vi "Find VI with Focus.vi"(8 "error in":errorcluster caption="error in (no error)", 9 "Exclude Callers":bool=TRUE caption="Exclude All Callers (T)", 10 "Exclude Levels":i32=-1 caption="Exclude Levels (call chain=-1)", 11 "Exclude Names":string[](array[string]) caption="Exclude Names (none)") -> (0 "error out":errorcluster, 1 "Changed?":bool, 2 "VI with Focus":refnum<vi>, 3 "Valid?":bool, 5 "VI Name":string)   [LabVIEW 2020]
doc: "Returns a reference to the frontmost VI panel. \n\nThis VI is reentrant (as indicated by the crosshatched background) so that references in use by one caller aren't closed by another. This also allows different callers to exclude different panels from consideration and to get a proper indication of whether a changed has occurred since their own last last call.\n\nThis is an enhancement of Jim Kring's Find Frontmost VI that returns a reference as well as a name, signals if this has changed since the last call, allows exclusion of VIs in the calling sequence of this VI or other VIs of the user's choice (useful for editing utilities that stay on top of all other windows), cleans up unused references, and runs, on average, 50 or more times faster.\n\nGenerates no errors.\n\nCopyright © 2003 by Paul F. Sullivan. All rights reserved. You are only permitted the usage indicated in your license agreement."
uses:
  TypeDefs/Find Focus State.ctl
panel:
  out "State Data":T2={"State"=enum."Excluded?", "Recent VI"=refnum, "Recent Number"=0, "Recent VI Name"="", "VI with Focus"=refnum, "Focus Number"=0, "Focus VI Name"="", "Valid?"=FALSE, "Changed?"=FALSE} {"Focus Number" format="%.0x"; "Recent Number" format="%.0x"}
  in  "State Data":T2={"State"=enum."Recent?", "Recent VI"=refnum, "Recent Number"=0, "Recent VI Name"="", "VI with Focus"=refnum, "Focus Number"=0, "Focus VI Name"="", "Valid?"=FALSE, "Changed?"=FALSE} {"Focus Number" format="%.0x"; "Recent Number" format="%.0x"}
  # "Find VI with Focus.vi\n\nReturns a reference to the frontmost VI panel.\n\nPlease visit http://www.OpenG.org to learn about the\nOpen Source LabVIEW software movement.\n\nNOTICE -- YOU MUST LEAVE THIS NOTICE IN PLACE.  PER THE TERMS OF THE LICENSE BELOW, YOU MAY SUBLICENSE THIS SOFTWARE \nIN ANY WAY THAT DOES NOT CONFLICT WITH THIS LICENSE.\n\n### BSD License (http://www.opensource.org/licenses/bsd-license.php) Begin ###\n \nCopyright (c) 2003, Paul F. Sullivan <Paul@SULLutions.com>\n\nAll rights reserved.\n\nRedistribution and use in source and binary forms, with or without modification, are permitted provided that the following conditions are met:\n\n    * Redistributions of source code must retain the above copyright notice, this list of conditions and the following disclaimer.\n    * Redistributions in binary form must reproduce the above copyright notice, this list of conditions and the following disclaimer in the \n       documentation and/or other materials provided with the distribution.\n    * Neither the name of SciWare, James Kring, Inc., nor the names of its contributors may be used to endorse or promote products derived \n       from this software without specific prior written permission.\n\nTHIS SOFTWARE IS PROVIDED BY THE COPYRIGHT HOLDERS AND CONTRIBUTORS \"AS IS\" AND ANY EXPRESS OR IMPLIED WARRANTIES, \nINCLUDING, BUT NOT LIMITED TO, THE IMPLIED WARRANTIES OF MERCHANTABILITY AND FITNESS FOR A PARTICULAR PURPOSE ARE \nDISCLAIMED. IN NO EVENT SHALL THE COPYRIGHT OWNER OR CONTRIBUTORS BE LIABLE FOR ANY DIRECT, INDIRECT, INCIDENTAL,\n SPECIAL, EXEMPLARY, OR CONSEQUENTIAL DAMAGES (INCLUDING, BUT NOT LIMITED TO, PROCUREMENT OF SUBSTITUTE GOODS OR \nSERVICES; LOSS OF USE, DATA, OR PROFITS; OR BUSINESS INTERRUPTION) HOWEVER CAUSED AND ON ANY THEORY OF LIABILITY, \nWHETHER IN CONTRACT, STRICT LIABILITY, OR TORT (INCLUDING NEGLIGENCE OR OTHERWISE) ARISING IN ANY WAY OUT OF THE USE \nOF THIS SOFTWARE, EVEN IF ADVISED OF THE POSSIBILITY OF SUCH DAMAGE.\n\n### BSD License End ###"
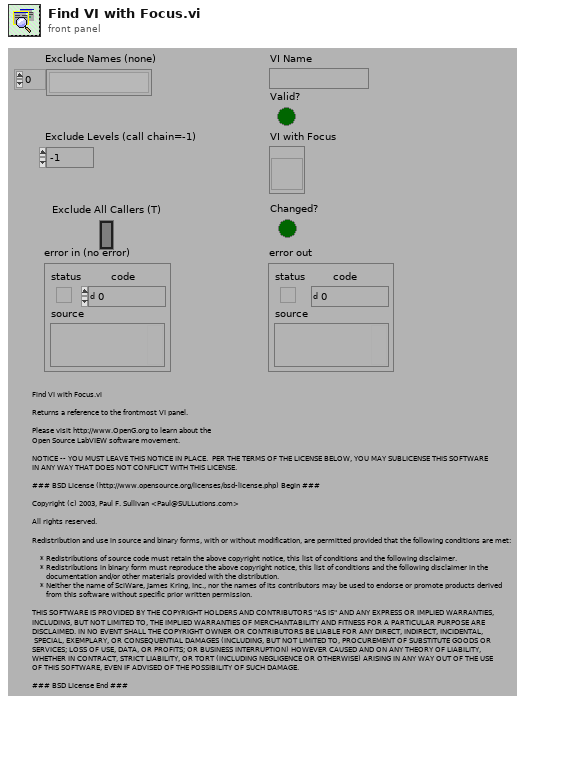
[diagram p1: front panel]
types:
  T1 = typedef "Find Focus State.ctl" = enum16{"Initialize", "Recent?", "Accepted?", "Excluded?", "VI Panel?", "Valid?", "Done"}
  T2 = cluster{"State":T1, "Recent VI":refnum<vi>, "Recent Number":u32, "Recent VI Name":string, "VI with Focus":refnum<vi>, "Focus Number":u32, "Focus VI Name":string, "Valid?":bool, "Changed?":bool}
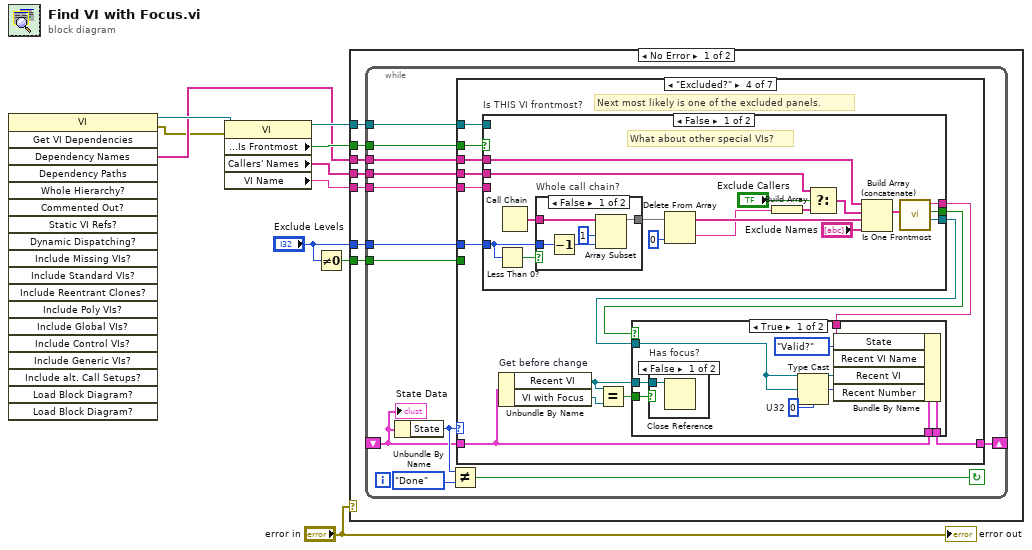
[diagram p0: block diagram]
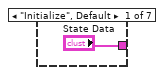
[diagram p2: hidden frame]
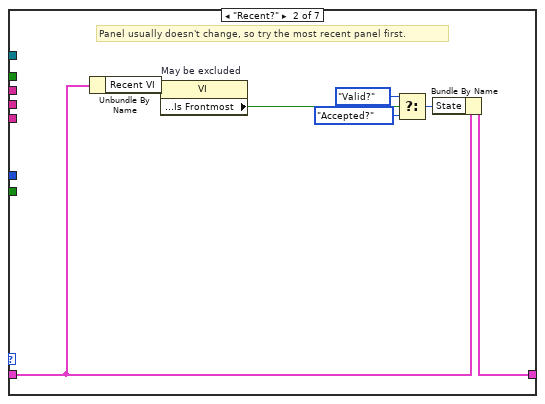
[diagram p3: hidden frame]
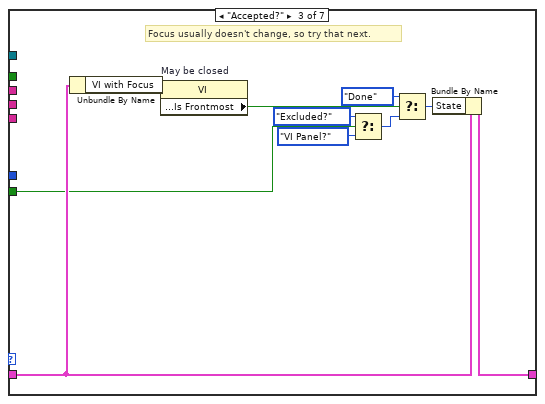
[diagram p4: hidden frame]
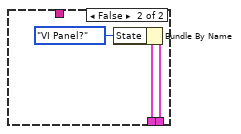
[diagram p6: hidden frame]
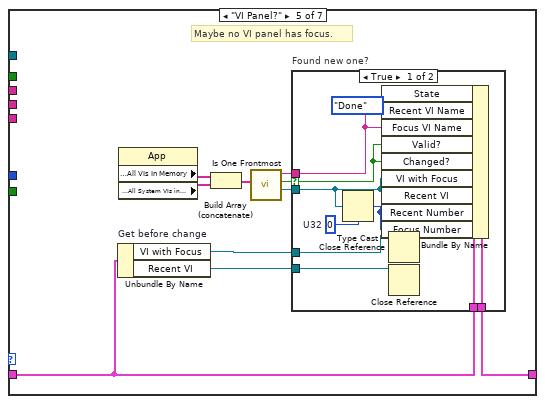
[diagram p9: hidden frame]
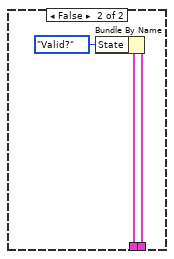
[diagram p10: hidden frame]
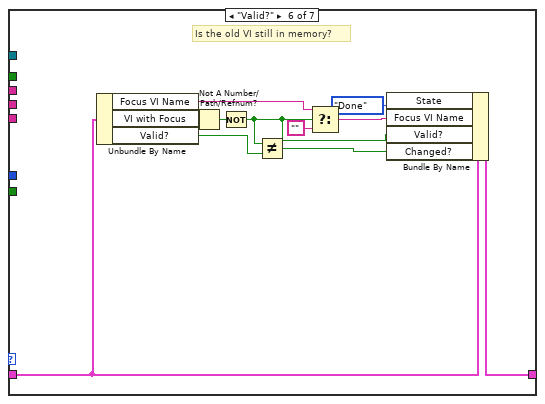
[diagram p11: hidden frame]
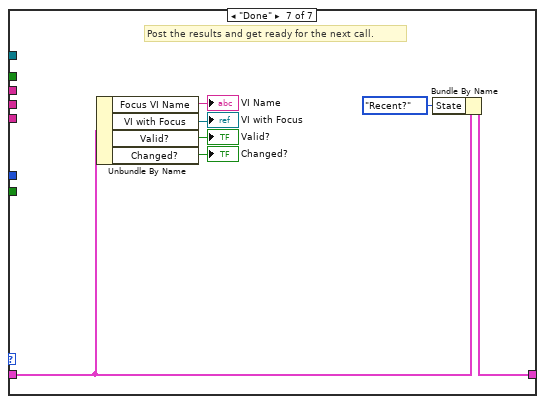
[diagram p12: hidden frame]
diagram:
  n1 = invoke class="VI" method="Get VI Dependencies"() -> (reference out=w3:refnum<vi>, error out=w1:errorcluster, "Dependency Names"=w2:string[])  [unwired: 19 in, 16 out]
  n2 = property class="VI"(reference=w3, error in=w1) -> (reference out=w7:refnum<vi>, "Front Panel Window:Is Frontmost"=w8:bool, "Callers' Names"=w9:string[], "VI Name"=w4:string)  [unwired: 1 out]
  n3 = Not Equal To 0?(x="Exclude Levels") -> (x != 0?=w5:bool)
  n4 = case shown="No Error" "error in" {
    tunnel: w9 -> [w17 _]
    tunnel: w2 -> [w16 _]
    tunnel: w8 -> [w15 _]
    tunnel: w7 -> [w14 _]
    tunnel: "Exclude Levels" -> [w13 _]
    tunnel: w5 -> [w12 _]
    tunnel: w4 -> [w11 _]
    frame No Error {
      n5 = while {
        tunnel: w11 -> [w19]
        tunnel: w12 -> [w21]
        tunnel: w13 -> [w22]
        tunnel: w14 -> [w20]
        tunnel: w15 -> [w23]
        tunnel: w16 -> [w24]
        tunnel: w17 -> [w25]
        shift-left: _ -> [w18]
        shift-right: [w27] -> _
        stop <- w26 continue-if-true
        n6 = Unbundle By Name(w18) -> ("State"=w28:T1)
        n7 = Not Equal?(x=w28, y=Find_Focus_State."Done" ("State")) -> (x != y?=w26:bool)
        n8 = case shown="\"Excluded?\"" w28 {
          tunnel: w23 -> [_ _ _ w61 _ _ _]
          tunnel: w25 -> [_ _ _ w60 _ _ _]
          tunnel: w24 -> [_ _ _ w59 _ _ _]
          tunnel: w22 -> [_ _ _ w58 _ _ _]
          tunnel: w21 -> [_ _ w39 _ _ _ _]
          tunnel: w18 -> [_ w36 w46 w51 w101 w131 w138]
          tunnel: ["State Data" w35 w45 w57 w106 w130 w137] -> w27
          tunnel: w20 -> [_ _ _ w54 _ _ _]
          tunnel: w19 -> [_ _ _ w52 _ _ _]
          frame "Initialize", Default {
          }
          frame "Recent?" {
            # "Panel usually doesn't change, so try the most recent panel first."
            n9 = Unbundle By Name(w36) -> ("Recent VI"=w37:refnum<vi>)
            n10 = property on="May be excluded" class="VI"(reference=w37) -> ("Front Panel Window:Is Frontmost"=w33:bool)  [unwired: 1 in, 2 out]
            n11 = Select(t=Find_Focus_State."Valid?" ("State"), s=w33, f=Find_Focus_State."Accepted?" ("State")) -> (s? t:f=w34:T1)
            n12 = Bundle By Name(cluster=w36, "State"=w34) -> (w35:T2)
          }
          frame "Accepted?" {
            # "Focus usually doesn't change, so try that next."
            n13 = Unbundle By Name(w46) -> ("VI with Focus"=w47:refnum<vi>)
            n14 = property on="May be closed" class="VI"(reference=w47) -> ("Front Panel Window:Is Frontmost"=w43:bool)  [unwired: 1 in, 2 out]
            n15 = Select(t=Find_Focus_State."Excluded?" ("State"), s=w39, f=Find_Focus_State."VI Panel?" ("State")) -> (s? t:f=w40:T1)
            n16 = Select(t=Find_Focus_State."Done" ("State"), s=w43, f=w40) -> (s? t:f=w44:T1)
            n17 = Bundle By Name(cluster=w46, "State"=w44) -> (w45:T2)
          }
          frame "Excluded?" {
            # "Next most likely is one of the excluded panels."
            n18 = case "Is THIS VI frontmost?" shown="False" w61 {
              selector: w61 -> [_ w100]
              tunnel: w58 -> [w78 _]
              tunnel: [w77 w100] -> w56
              tunnel: w60 -> [w87 _]
              tunnel: w59 -> [w82 _]
              tunnel: [w76 w99] -> w55
              tunnel: w54 -> [_ w99]
              tunnel: [w75 w98] -> w53
              tunnel: w52 -> [_ w98]
              frame False {
                # "What about other special VIs?"
                n19 = Less Than 0?(x=w78) -> (x < 0?=w89:bool)
                n20 = Call Chain() -> (call chain=w90:string[])
                n21 = case "Whole call chain?" shown="False" w89 {
                  tunnel: w78 -> [w96 _]
                  tunnel: [w93 w97] -> w86
                  tunnel: w90 -> [w92 w97]
                  frame False {
                    n22 = Decrement(x=w96) -> (x-1=w94:i32)
                    n23 = Array Subset(array=w92, index=1 ("Array Index"), length=w94) -> (w93:string[])
                  }
                  frame True {
                  }
                }
                n24 = Delete From Array(array=w86, index=0 ("Index")) -> (deleted portion=w84:string, array with subset deleted=w88:string[])  [unwired: 1 in]
                n25 = Build Array(w84) -> (w83:string[])
                n26 = Select(t=w87, s="Exclude Callers", f=w83) -> (s? t:f=w81:string[])
                n27 = Build Array (concatenate)(w82, w81, w88, "Exclude Names") -> (w91:string[])
                n28 = call "Is One Frontmost.vi"("VI names"=w91) -> ("VI Refnum"=w76:refnum<vi>, "yes"=w77:bool, "VI name"=w75:string)  [unwired: 7 in, 1 out]
              }
              frame True {
              }
            }
            n29 = Unbundle By Name "Get before change"(w51) -> ("Recent VI"=w49:refnum<vi>, "VI with Focus"=w50:refnum<vi>)
            n30 = Equal?(x=w49, y=w50) -> (x = y?=w48:bool)
            n31 = case shown="True" w56 {
              tunnel: [w70 w74] -> w57
              tunnel: w51 -> [w69 w73]
              tunnel: w55 -> [w65 _]
              tunnel: w49 -> [w67 _]
              tunnel: w53 -> [w62 _]
              tunnel: w48 -> [w63 _]
              frame True {
                w64 = u32 0  # U32
                n32 = case "Has focus?" shown="False" w63 {
                  tunnel: w67 -> [w71 _]
                  frame False {
                    n33 = Close Reference(reference=w71) -> ()  [unwired: 1 in, 1 out]
                  }
                  frame True {
                  }
                }
                n34 = Type Cast(type=w64, x=w65) -> (*(type *) &x=w66:u32)
                n35 = Bundle By Name(cluster=w69, "State"=Find_Focus_State."Valid?", "Recent VI Name"=w62, "Recent VI"=w65, "Recent Number"=w66) -> (w70:T2)
              }
              frame False {
                n36 = Bundle By Name(cluster=w73, "State"=Find_Focus_State."VI Panel?") -> (w74:T2)
              }
            }
          }
          frame "VI Panel?" {
            # "Maybe no VI panel has focus."
            n37 = Unbundle By Name "Get before change"(w101) -> ("VI with Focus"=w103:refnum<vi>, "Recent VI"=w102:refnum<vi>)
            n38 = property class="App"() -> ("Application:All VIs In Memory"=w110:string[], "Application:All System VIs in Memory"=w109:string[])  [unwired: 2 in, 2 out]
            n39 = Build Array (concatenate)(w110, w109) -> (w108:string[])
            n40 = call "Is One Frontmost.vi"("VI names"=w108) -> ("VI Refnum"=w104:refnum<vi>, "yes"=w107:bool, "VI name"=w105:string)  [unwired: 7 in, 1 out]
            n41 = case "Found new one?" shown="True" w107 {
              selector: w107 -> [w118 _]
              tunnel: w101 -> [w120 w123]
              tunnel: [w119 w122] -> w106
              tunnel: w105 -> [w116 _]
              tunnel: w104 -> [w112 _]
              tunnel: w103 -> [w114 _]
              tunnel: w102 -> [w115 _]
              frame True {
                w113 = u32 0  # U32
                n42 = Type Cast(type=w113, x=w112) -> (*(type *) &x=w111:u32)
                n43 = Bundle By Name(cluster=w120, "State"=Find_Focus_State."Done", "Recent VI Name"=w116, "Focus VI Name"=w116, "Valid?"=w118, "Changed?"=w118, "VI with Focus"=w112, "Recent VI"=w112, "Recent Number"=w111, "Focus Number"=w111) -> (w119:T2)
                n44 = Close Reference(reference=w114) -> ()  [unwired: 1 in, 1 out]
                n45 = Close Reference(reference=w115) -> ()  [unwired: 1 in, 1 out]
              }
              frame False {
                n46 = Bundle By Name(cluster=w123, "State"=Find_Focus_State."Valid?") -> (w122:T2)
              }
            }
          }
          frame "Valid?" {
            # "Is the old VI still in memory?"
            n47 = Unbundle By Name(w131) -> ("Focus VI Name"=w126:string, "VI with Focus"=w134:refnum<vi>, "Valid?"=w132:bool)
            n48 = Not A Number/Path/Refnum?(number/path/refnum=w134) -> (NaN/Path/Refnum?=w133:bool)
            n49 = Not(x=w133) -> (.not. x?=w125:bool)
            n50 = Not Equal?(x=w125, y=w132) -> (x != y?=w129:bool)
            n51 = Select(t=w126, s=w125, f="") -> (s? t:f=w128:string)
            n52 = Bundle By Name(cluster=w131, "State"=Find_Focus_State."Done", "Focus VI Name"=w128, "Valid?"=w125, "Changed?"=w129) -> (w130:T2)
          }
          frame "Done" {
            # "Post the results and get ready for the next call."
            n53 = Unbundle By Name(w138) -> ("Focus VI Name"=→"VI Name":string, "VI with Focus"=→"VI with Focus":refnum<vi>, "Valid?"=→"Valid?":bool, "Changed?"=→"Changed?":bool)
            n54 = Bundle By Name(cluster=w138, "State"=Find_Focus_State."Recent?") -> (w137:T2)
          }
        }
        "State Data" <- w18
      }
    }
    frame Error {
    }
  }
  "error out" <- "error in"
